vi "TEST.vi"() -> ()   [LabVIEW 2019]
uses:
  <userlib>/Haptic Prog Interface/Haptic Prog Interface.lvlib
panel:
  in  "Minimum Force":T1={"Fx (N)"=-3.0, "Fy (N)"=-3.0, "Fz (N)"=-3.0} {"Fx (N)" format="%.1f"; "Fy (N)" format="%.1f"; "Fz (N)" format="%.1f"}
  in  "Maximum Force":T1={"Fx (N)"=3.0, "Fy (N)"=3.0, "Fz (N)"=3.0} {"Fx (N)" format="%.1f"; "Fy (N)" format="%.1f"; "Fz (N)" format="%.1f"}
  out "Button State":bool
  in  "Drag Coefficients":T2={"kx (N/m)"=0.001, "ky (N/m)"=0.001, "kz (N/m)"=0.001}
  in  "Drag Force Toggles":T3={"X Drag"=TRUE, "Y Drag"=TRUE, "Z Drag"=TRUE}
  in  "Wall Stiffness":dbl=0.2
  in  "Restrict to Frame":bool=TRUE
  in  "Forces Write":T1
  in  "Mode Selection":u16(ring) items=["Custom Mode", "Read Mode", "STM Write Mode", "AFM Write Mode"]
  out "Position (Reframed)":cluster{"x (m)":dbl, "y (m)":dbl, "z (mm)":dbl} {"z (mm)" format="%.1f"; "y (m)" format="%.1p"; "x (m)" format="%.1p"}
  in  "Frame Properties":T4={"X Origin (m)"=0.0, "Y Origin (m)"=0.0, "FW (m)"=1e-09, "FH (m)"=1e-09}
  out "Velocity":T5 {"vz (mm/s)" format="%.1f"; "vy (mm/s)" format="%.1f"; "vx (mm/s)" format="%.1f"}
  out "Forces":T1 {"Fz (N)" format="%.1f"; "Fy (N)" format="%.1f"; "Fx (N)" format="%.1f"}
  out "Angles":cluster{"theta":dbl, "phi":dbl, "psi":dbl} {"psi" format="%.1f"; "phi" format="%.1f"; "theta" format="%.1f"}
  out "Position":T6 {"z (mm)" format="%.1p"; "y (mm)" format="%.1p"; "x (mm)" format="%.1p"}
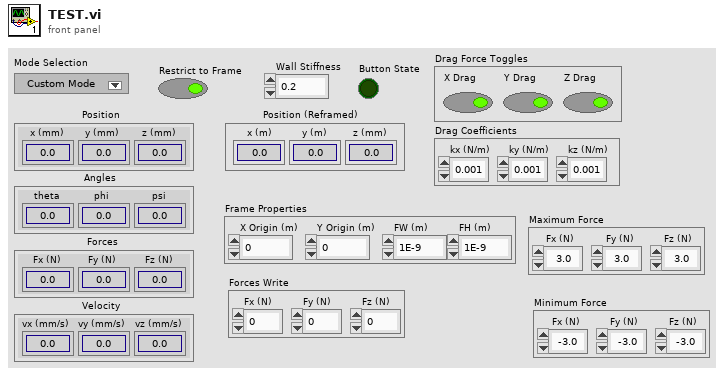
[diagram p1: front panel]
types:
  T1 = cluster{"Fx (N)":dbl, "Fy (N)":dbl, "Fz (N)":dbl}
  T2 = cluster{"kx (N/m)":dbl, "ky (N/m)":dbl, "kz (N/m)":dbl}
  T3 = cluster{"X Drag":bool, "Y Drag":bool, "Z Drag":bool}
  T4 = cluster{"X Origin (m)":dbl, "Y Origin (m)":dbl, "FW (m)":dbl, "FH (m)":dbl}
  T5 = cluster{"vx (mm/s)":dbl, "vy (mm/s)":dbl, "vz (mm/s)":dbl}
  T6 = cluster{"x (mm)":dbl, "y (mm)":dbl, "z (mm)":dbl}
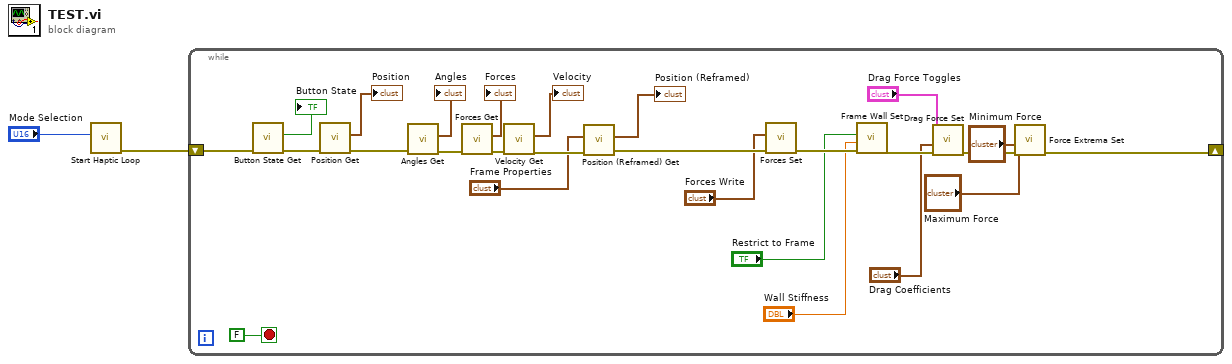
[diagram p0: block diagram]
diagram:
  n1 = call <userlib>:"Start Haptic Loop.vi"("Mode Selection"="Mode Selection") -> ("error out"=w2:errorcluster)  [unwired: 10 in]
  n2 = while {
    shift-right: [w5] -> _
    shift-left: w2 -> [w27]
    stop <- FALSE stop-if-true
    n3 = call <userlib>:"Button State Get.vi"("error in (no error)"=w27) -> ("error out"=w26:errorcluster, "Button State"=→"Button State":bool)  [unwired: 9 in]
    n4 = call <userlib>:"Position Get.vi"("error in (no error)"=w26) -> ("error out"=w24:errorcluster, "Position"=→"Position":T6)  [unwired: 9 in]
    n5 = call <userlib>:"Angles Get.vi"("error in (no error)"=w24) -> ("error out"=w23:errorcluster, "Angles"=→"Angles":cluster{"theta":dbl, "phi":dbl, "psi":dbl})  [unwired: 9 in]
    n6 = call <userlib>:"Forces Get.vi"("error in (no error)"=w23) -> ("error out"=w22:errorcluster, "Forces"=→"Forces":T1)  [unwired: 9 in]
    n7 = call <userlib>:"Velocity Get.vi"("error in (no error)"=w22) -> ("error out"=w18:errorcluster, "Velocity"=→"Velocity":T5)  [unwired: 9 in]
    n8 = call <userlib>:"Position (Reframed) Get.vi"("error in (no error)"=w18, "Frame Properties"="Frame Properties") -> ("error out"=w15:errorcluster, "Position (Reframed)"=→"Position (Reframed)":cluster{"x (m)":dbl, "y (m)":dbl, "z (mm)":dbl})  [unwired: 8 in]
    n9 = call <userlib>:"Forces Set.vi"("error in (no error)"=w15, "Forces"="Forces Write") -> ("error out"=w13:errorcluster)  [unwired: 9 in]
    n10 = call <userlib>:"Frame Wall Set.vi"("error in (no error)"=w13, "Wall Stiffness"="Wall Stiffness", "Restrict to Frame"="Restrict to Frame") -> ("error out"=w10:errorcluster)  [unwired: 8 in]
    n11 = call <userlib>:"Drag Force Set.vi"("error in (no error)"=w10, "Drag Coefficients"="Drag Coefficients", "Drag Force Toggles"="Drag Force Toggles") -> ("error out"=w6:errorcluster)  [unwired: 8 in]
    n12 = call <userlib>:"Force Extrema Set.vi"("error in (no error)"=w6, "Minimum Force"="Minimum Force", "Maximum Force"="Maximum Force") -> ("error out"=w5:errorcluster)  [unwired: 8 in]
  }
